vi "Created Events.vi"(8 "Created Event Alias":string, 9 "Priority?":bool, 10 "Msg Strategy":refnum<class "Msg Strategy.lvclass">, 11 "Queue jettl in":refnum<class "Queue jettl.lvclass">) -> (3 "Queue jettl out":refnum<class "Queue jettl.lvclass">)   [LabVIEW 2021, in "jettl.lvlib" / "Queue jettl.lvclass"]
uses:
  Queue jettl.lvclass
  Msg Strategy/Msg Strategy.lvclass
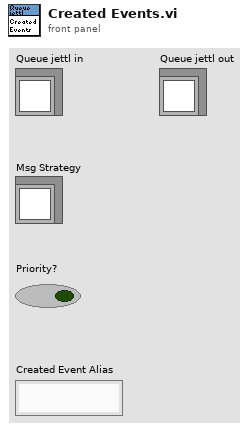
[diagram p1: front panel]
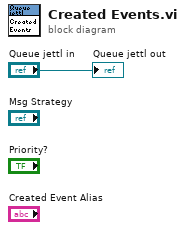
[diagram p0: block diagram]
diagram:
  "Queue jettl out" <- "Queue jettl in"
